vi "get Texture Pixels.vi"(11 "Texture Name":string) -> (3 "Pixels":u32[][](array[numeric]))   [LabVIEW 2021, in "Resource Manager.lvclass"]
uses:
  Resource Manager.lvclass
  Resource Manager.lvclass/Resource Manager.ctl
  Globals.vi
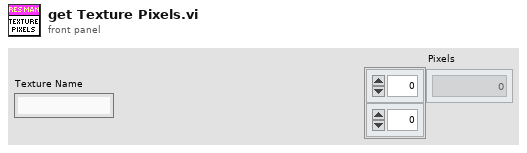
[diagram p1: front panel]
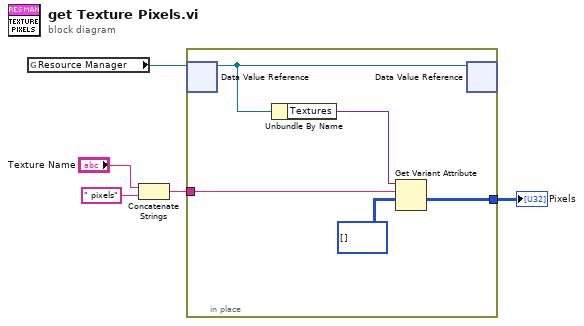
[diagram p0: block diagram]
diagram:
  n1 = global read "Globals.vi" "Resource Manager"() -> (w4:refnum<data-value>)
  n2 = Concatenate Strings("Texture Name", " pixels" ("string")) -> (w1:string)
  n3 = in-place {
    in-place-border: w1 -> [w10]
    in-place-border: [w9] -> w5
    n4 = in-place-dvr #1(w4) -> (w7:refnum<class "Resource Manager.lvclass">)  [unwired: 1 out]
    n5 = Unbundle By Name(w7) -> ("Textures"=w8:variant)
    n6 = Get Variant Attribute(Variant=w8, name=w10, default value (empty Variant)=u32[][] [] ("Pixels")) -> (value=w9:u32[][])  [unwired: 1 in, 3 out]
    n7 = in-place-dvr #1(w7) -> ()  [unwired: 2 out]
  }
  "Pixels" <- w5
